vi "automatic_start.vi"(8 "error in (no error)":errorcluster, 10 "data":variant, 11 "criteria":variant) -> (0 "error out":errorcluster)   [LabVIEW 2015, in "lv-recipe-machine.lvlib"]
doc: "automatic_start.vi can be used to start a given recipe with an optional criteria. When executed successfully, the internal recipe_logic will change the automatic state to running which will start executing the configured recipe."
uses:
  lv-recipe-machine.lvlib
  _controls/error.ctl
  private/_controls/timers.ctl
  _controls/automatic_state.ctl
  private/_controls/timer_command.ctl
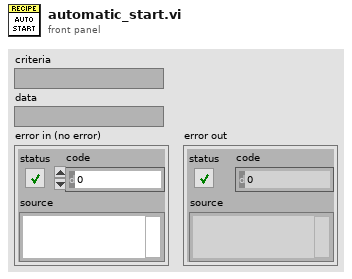
[diagram p1: front panel]
types:
  T1 = typedef "lv-recipe-machine.lvlib/timers.ctl" = enum16{"<timers>", "step", "recipe", "<null>"}
  T2 = typedef "lv-recipe-machine.lvlib/error.ctl" = enum16{"<error>", "bad_command", "command_queue_timeout", "stop_notifier_timeout", "die_command_timeout", "not_in_manual_mode", "not_in_automatic_mode", "not_in_automatic_idle", "not_in_automatic_running", "not_in_automatic_paused", "automatic_step_not_found", "manual_action_not_found", "automatic_not_transition_vi", "transition_step_not_found", "unsupported_vi_type", "<null>"}
  T3 = typedef "lv-recipe-machine.lvlib/automatic_state.ctl" = enum16{"<automatic_state>", "failed", "idle", "running", "paused", "stopped", "<null>"}
  T4 = typedef "lv-recipe-machine.lvlib/timer_command.ctl" = enum16{"<timer_command>", "start", "read", "pause", "resume", "stop", "<null>"}
  T5 = typedef "lv-recipe-machine.lvlib/references.ctl" = cluster{"semaphore":T6, "input_queue":refnum<queue>, "output_queue":refnum<queue>, "transition_queue":refnum<queue>, "data_dvr":refnum<data-value>, "stop_notifier":refnum<notifier>, "change_in_event":refnum<user-event>, "change_out_event":refnum<user-event>, "status_event":refnum<user-event>}
  T6 = typedef "Semaphore RefNum" = refnum<k1>
  T7 = typedef "lv-recipe-machine.lvlib/data.ctl" = cluster{"configuration":T8, "working":cluster{"recipe_data":T9}}
  T8 = typedef "lv-recipe-machine.lvlib/configuration.ctl" = cluster{"change_in_timeout_ms":i32}
  T9 = typedef "lv-recipe-machine.lvlib/recipe_data.ctl" = cluster{"mode":T10, "manual_state":T11, "automatic_state":T3, "previous_automatic_state":T3, "error":errorcluster, "timer []":T12[], "manual":cluster{"step_action":string, "data":variant, "actions":variant}, "automatic":cluster{"data":variant, "steps":variant, "criteria":variant, "transition":string, "index":i32, "step_launched":bool, "recipe []":T13[]}}
  T10 = typedef "lv-recipe-machine.lvlib/mode.ctl" = enum16{"<mode>", "manual", "automatic", "<null>"}
  T11 = typedef "lv-recipe-machine.lvlib/manual_state.ctl" = enum16{"<manual_state>", "failed", "action", "running", "idle", "<null>"}
  T12 = typedef "lv-recipe-machine.lvlib/timer.ctl" = cluster{"elapsed_time":dbl, "previous_time":dbl}
  T13 = typedef "lv-recipe-machine.lvlib/recipe_step.ctl" = cluster{"step":string, "data":variant}
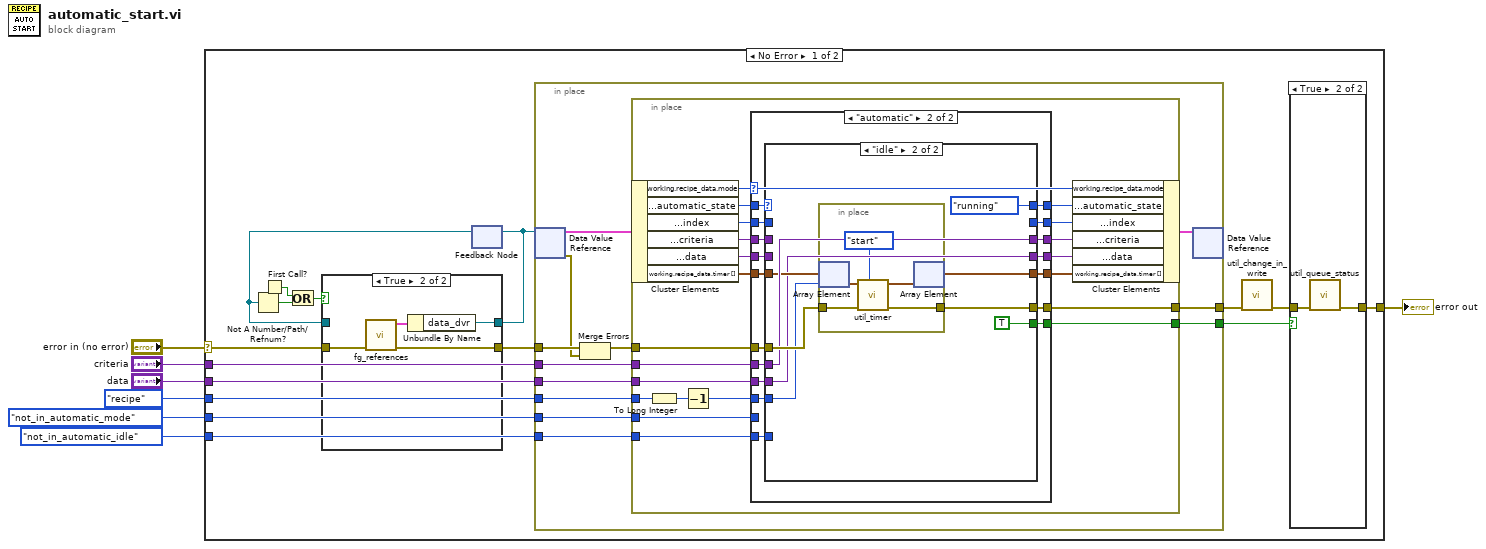
[diagram p0: block diagram]
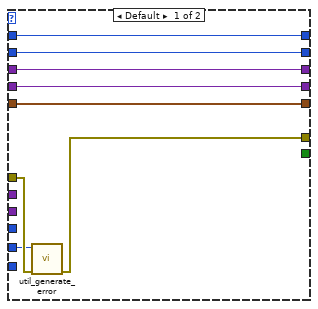
[diagram p3: hidden frame]
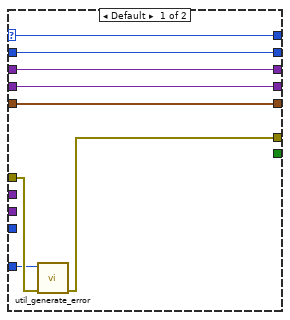
[diagram p4: hidden frame]
diagram:
  n1 = case shown="No Error" "error in (no error)" {
    selector: "error in (no error)" -> [w10 w113]
    tunnel: [w18 w113] -> w6
    tunnel: "criteria" -> [w23 _]
    tunnel: error."not_in_automatic_mode" ("error") -> [w22 _]
    tunnel: error."not_in_automatic_idle" ("error") -> [w21 _]
    tunnel: timers."recipe" ("timers") -> [w16 _]
    tunnel: "data" -> [w8 _]
    frame No Error {
      n2 = First Call?() -> (First Call?: T/F=w14:bool)
      n3 = feedback #1() -> (w13:refnum<data-value>)  [unwired: 1 in]
      n4 = Not A Number/Path/Refnum?(number/path/refnum=w13) -> (NaN/Path/Refnum?=w15:bool)
      n5 = Or(x=w14, y=w15) -> (x .or. y?=w12:bool)
      n6 = case shown="True" w12 {
        tunnel: w10 -> [w24 w29]
        tunnel: [w24 w28] -> w9
        tunnel: [w25 w26] -> w11
        tunnel: w13 -> [w25 _]
        frame False {
        }
        frame True {
          n7 = call "fg_references.vi"("error in (no error)"=w29) -> ("error out"=w28:errorcluster, "references out"=w27:T5)  [unwired: 9 in]
          n8 = Unbundle By Name(w27) -> ("data_dvr"=w26:refnum<data-value>)
        }
      }
      n9 = feedback-in #1(w11) -> ()
      n10 = in-place {
        in-place-border: w9 -> [w41]
        in-place-border: w23 -> [w36]
        in-place-border: w22 -> [w35]
        in-place-border: [w34] -> w19
        in-place-border: w21 -> [w33]
        in-place-border: [w32] -> w17
        in-place-border: w16 -> [w31]
        in-place-border: w8 -> [w30]
        n11 = in-place-dvr #2(w11) -> (w39:T7, w40:errorcluster)
        n12 = Merge Errors(w41, w40) -> (w38:errorcluster)
        n13 = in-place {
          in-place-border: w38 -> [w59]
          in-place-border: w36 -> [w58]
          in-place-border: w35 -> [w57]
          in-place-border: [w56] -> w34
          in-place-border: w33 -> [w51]
          in-place-border: [w50] -> w32
          in-place-border: w31 -> [w47]
          in-place-border: w30 -> [w44]
          n14 = in-place-cluster #3(w39) -> ("working.recipe_data.mode"=w55:T10, "working.recipe_data.automatic_state"=w62:T3, "working.recipe_data.automatic.index"=w61:i32, "working.recipe_data.automatic.criteria"=w60:variant, "working.recipe_data.automatic.data"=w43:variant, "working.recipe_data.timer []"=w49:T12[])
          n15 = To Long Integer(number=w47) -> (32bit integer=w45:i32)
          n16 = Decrement(x=w45) -> (x-1=w46:i32)
          n17 = case shown="\"automatic\"" w55 {
            tunnel: w62 -> [w67 w86]
            tunnel: w61 -> [w66 w85]
            tunnel: w60 -> [w65 w82]
            tunnel: w59 -> [w70 w84]
            tunnel: w58 -> [_ w78]
            tunnel: w57 -> [w69 _]
            tunnel: [w68 w83] -> w56
            tunnel: [w67 w79] -> w54
            tunnel: [w66 w80] -> w53
            tunnel: [w65 w81] -> w52
            tunnel: w51 -> [_ w87]
            tunnel: [_ w77] -> w50
            tunnel: w49 -> [w64 w76]
            tunnel: [w64 w75] -> w48
            tunnel: w46 -> [_ w74]
            tunnel: w44 -> [_ w73]
            tunnel: w43 -> [w63 w72]
            tunnel: [w63 w71] -> w42
            frame Default {
              n18 = call "util_generate_error.vi"("error in (no error)"=w70, "error"=w69) -> ("error out"=w68:errorcluster)  [unwired: 9 in]
            }
            frame "automatic" {
              n19 = case shown="\"idle\"" w86 {
                selector: w86 -> [w90 _]
                tunnel: w87 -> [w93 _]
                tunnel: w85 -> [w91 _]
                tunnel: w84 -> [w95 w104]
                tunnel: [w94 w97] -> w83
                tunnel: w82 -> [w92 _]
                tunnel: [w92 w102] -> w81
                tunnel: [w91 _] -> w80
                tunnel: [w90 automatic_state."running" ("automatic_state")] -> w79
                tunnel: w78 -> [_ w102]
                tunnel: [_ TRUE] -> w77
                tunnel: w76 -> [w89 w100]
                tunnel: [w89 w99] -> w75
                tunnel: w74 -> [_ w98]
                tunnel: w73 -> [_ w96]
                tunnel: w72 -> [w88 _]
                tunnel: [w88 w96] -> w71
                frame Default {
                  n20 = call "util_generate_error.vi"("error in (no error)"=w95, "error"=w93) -> ("error out"=w94:errorcluster)  [unwired: 9 in]
                }
                frame "idle" {
                  n21 = in-place {
                    in-place-border: w104 -> [w106]
                    in-place-border: [w105] -> w97
                    n22 = in-place-array #4(w100, w98) -> (w108:T12)
                    n23 = call "util_timer.vi"("timer_command"=timer_command."start", "error in (no error)"=w106, "timer in"=w108) -> ("error out"=w105:errorcluster, "timer out"=w107:T12)  [unwired: 6 in, 1 out]
                    n24 = in-place-array #4(w107) -> (w99:T12[])  [unwired: 1 out]
                  }
                }
              }
            }
          }
          n25 = in-place-cluster #3("working.recipe_data.mode"=w55, "working.recipe_data.automatic_state"=w54, "working.recipe_data.automatic.index"=w53, "working.recipe_data.automatic.criteria"=w52, "working.recipe_data.automatic.data"=w42, "working.recipe_data.timer []"=w48) -> (w37:T7)
        }
        n26 = in-place-dvr #2(w37) -> ()  [unwired: 2 out]
      }
      n27 = call "util_change_in_write.vi"("error in (no error)"=w19) -> ("error out"=w20:errorcluster)  [unwired: 10 in]
      n28 = case shown="True" w17 {
        tunnel: w20 -> [w110 w112]
        tunnel: [w110 w111] -> w18
        frame False {
        }
        frame True {
          n29 = call "util_queue_status.vi"("error in (no error)"=w112) -> ("error out"=w111:errorcluster)  [unwired: 10 in]
        }
      }
    }
    frame Error {
    }
  }
  "error out" <- w6
